vi "Write Comparison type.vi"(9 "Comparison type":T1, 11 "CItemMatch in":refnum<class "CItemMatch.lvclass">) -> (3 "CItemMatch out":refnum<class "CItemMatch.lvclass">)   [LabVIEW 2020, in "DependencyInspection.lvlib" / "CItemMatch.lvclass"]
uses:
  CItemMatch.lvclass
  TypeDefs/ComparisonType.ctl
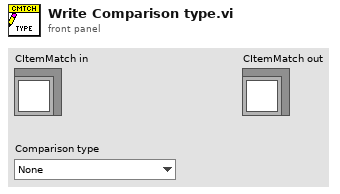
[diagram p1: front panel]
types:
  T1 = typedef "DependencyInspection.lvlib/CItemMatch.lvclass/ComparisonType.ctl" = enum16{"None", "Ends with", "Equals", "Not equal", "Starts with", "Contains", "Matches pattern"}
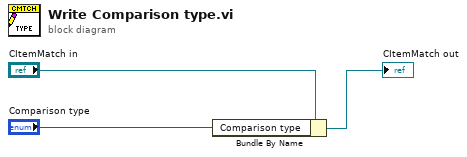
[diagram p0: block diagram]
diagram:
  n1 = Bundle By Name(cluster="CItemMatch in", "Comparison type"="Comparison type") -> (→"CItemMatch out":refnum<class "CItemMatch.lvclass">)
